vi "Comma Separated Pin Names.vi"(0 "Pin Names":string[](array[string]), 5 "error in (no error)":errorcluster) -> (4 "PinNames OUT":string, 6 "error out":errorcluster)   [LabVIEW 2024, in "devicePowerSequencerCoreLogic.lvlib"]
uses:
  devicePowerSequencerCoreLogic.lvlib
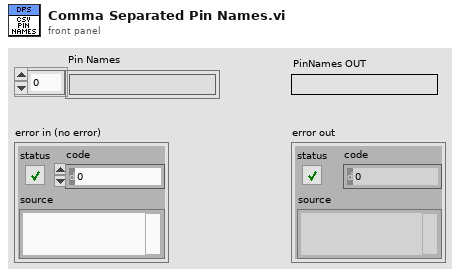
[diagram p1: front panel]
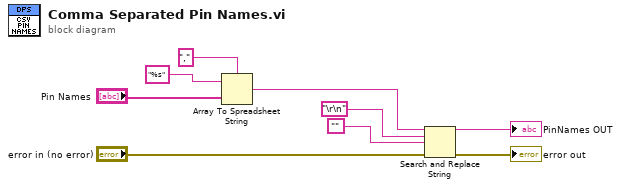
[diagram p0: block diagram]
diagram:
  n1 = Array To Spreadsheet String(delimiter (Tab)=",", array="Pin Names", 3:"%s" ("format string")) -> (spreadsheet string=w9:string)
  n2 = Search and Replace String(input string=w9, search string="\r\n", replace string="", error in="error in (no error)") -> (result string=→"PinNames OUT":string, error out=→"error out":errorcluster)  [unwired: 4 in, 2 out]
